vi "Read Brake On.vi"(8 "error in (no error)":errorcluster, 11 "Elevator in":refnum<class "Elevator.lvclass">) -> (0 "error out":errorcluster, 2 "Brake On":bool, 3 "Elevator out":refnum<class "Elevator.lvclass">)   [LabVIEW 2014, in "Elevator.lvlib" / "Elevator.lvclass"]
uses:
  Elevator.lvclass
  Elevator.lvclass/Elevator.ctl
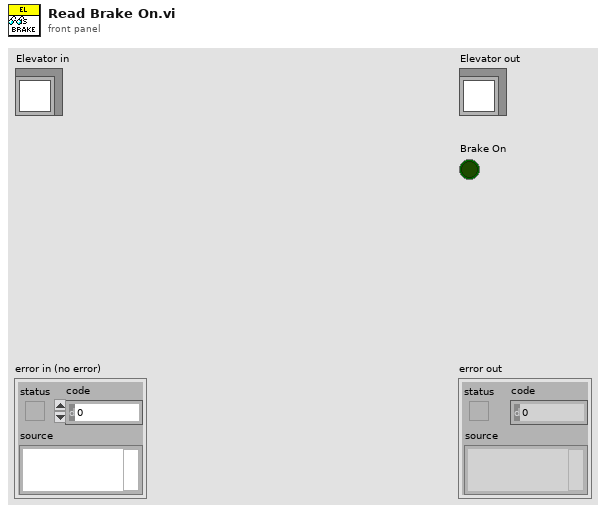
[diagram p1: front panel]
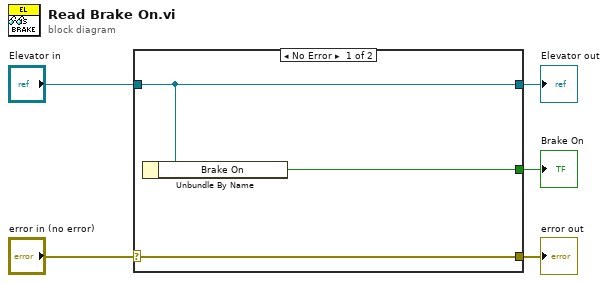
[diagram p0: block diagram]
diagram:
  n1 = case shown="No Error" "error in (no error)" {
    selector: "error in (no error)" -> [w8 w9]
    tunnel: [w8 w9] -> w4
    tunnel: [w7 w10] -> w2
    tunnel: "Elevator in" -> [w7 w10]
    tunnel: [w6 _] -> w1
    frame No Error {
      n2 = Unbundle By Name(w7) -> ("Brake On"=w6:bool)
    }
    frame Error {
    }
  }
  "error out" <- w4
  "Elevator out" <- w2
  "Brake On" <- w1
